vi "Riccati_Check_Detectable.vi"(9 "Q":T1, 11 "A":T1) -> (3 "Bad":bool)   [LabVIEW 2019, in "Trajectory_Library.lvlib"]
uses:
  <vilib>/Analysis/Matrix/Datatypes/RealMatrix.ctl
  Trajectory_Library.lvlib
  <vilib>/Analysis/Matrix/NI_Matrix.lvlib
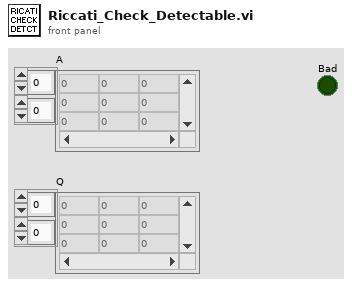
[diagram p1: front panel]
types:
  T1 = typedef "NI_Matrix.lvlib/RealMatrix.ctl" = dbl[][]
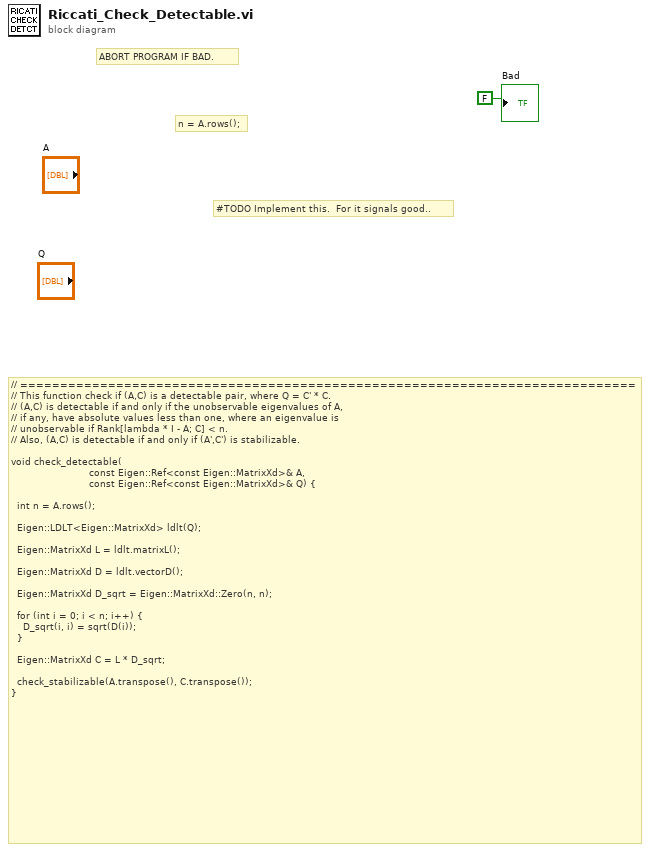
[diagram p0: block diagram]
diagram:
  # "#TODO Implement this.  For it signals good.."
  # "n = A.rows();"
  # "// =============================================================================\n// This function check if (A,C) is a detectable pair, where Q = C' * C.\n// (A,C) is detectable if and only if the unobservable eigenvalues of A,\n// if any, have absolute values less than one, where an eigenvalue is\n// unobservable if Rank[lambda * I - A; C] < n.\n// Also, (A,C) is detectable if and only if (A',C') is stabilizable.\n\nvoid check_detectable(\n                          const Eigen::Ref<const Eigen::MatrixXd>& A,\n                          const Eigen::Ref<const Eigen::MatrixXd>& Q) {\n\n  int n = A.rows();\n\n  Eigen::LDLT<Eigen::MatrixXd> ldlt(Q);\n\n  Eigen::MatrixXd L = ldlt.matrixL();\n\n  Eigen::MatrixXd D = ldlt.vectorD();\n\n  Eigen::MatrixXd D_sqrt = Eigen::MatrixXd::Zero(n, n);\n\n  for (int i = 0; i < n; i++) {\n    D_sqrt(i, i) = sqrt(D(i));\n  }\n\n  Eigen::MatrixXd C = L * D_sqrt;\n\n  check_stabilizable(A.transpose(), C.transpose());\n}"
  # "ABORT PROGRAM IF BAD."
  "Bad" <- FALSE
